vi "Multi_moments_LDA+_An.vi"(3 "Timescales":dbl[](array[numeric]), 4 "Measurement top level?":bool, 6 "Vari Spaced":dbl[][](array[numeric]) format="%.2f") -> (0 "Max Measurement time up":bool, 1 "File info":string[](array[string]), 2 "Vel stat display":string[][](table))   [LabVIEW 2010]
uses:
  Controls/Post_Process.ctl
  Controls/User_Specific_mode.ctl
  Globals/Meas_global.vi
  Globals/Trav_pos_global.vi
  Globals/Dynamic_call_global.ph.vi
  Globals/LDA_meas_global_1.vi
  Acquisition/PWA/PWAtasksGLOBAL.vi
panel:
  out "Sd Error Theshold value":dbl
  out "Instrument Code Name":string
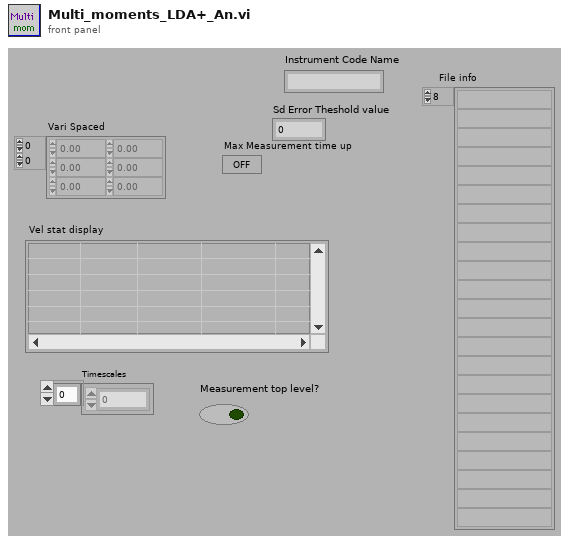
[diagram p1: front panel]
types:
  T1 = typedef "Analysis_info_cluster.ctl" = cluster{"Colour":u32, "Inst type":T2, "Inst name":string, "Symbol":string, "Code name":string, "Extra Info":string, "Inst Array":T3, "Index":i32, "Voltage Index":i32, "Extra Titles":string[], "Extra Values":string[]}
  T2 = typedef "Inst_type.ctl" = enum16{"Propeller anemometer", "Raw voltage", "Pressure Transducer", "Pitot-static tube", "Preston tube", "Hot wire", "Cross wire 1", "Cross wire 2", "Generic Linear", "Generic Polynomial", "Generic BackPoly", "Fast FID", "Thermocouple", "Cold wire", "Pulsed Wire", "LDA Vel", "LDA Tran time", "LDA Arr time"}
  T3 = typedef "Instrument_Array.ctl" = enum16{"PWA", "LDA", "Analogue"}
  T4 = typedef "Post_Process.ctl" = enum16{"Take New Data", "Post Process Raw Data File"}
  T5 = typedef "PWA_Data.ctl" = enum16{"No PWA Data", "One Ch PWA"}
  T6 = typedef "User_Specific_mode.ctl" = enum16{"Check VI only", "Run VI"}
  T7 = cluster{"Name":string, "X":dbl, "Y":dbl, "Z":dbl}[]
  T8 = typedef "Traverse_cluster.ctl" = cluster{"Start X":dbl, "Start Y":dbl, "Start Z":dbl, "End X":dbl, "End Y":dbl, "End Z":dbl, "No. of pts.":i32, "Spacing":T9, "Filename":path, "Tunnel Speed":dbl, "Averaging time (min)":dbl, "Extra Commands":string, "Specific Arguments":string, "Emission Rate (l/min)":dbl, "Trace Gas Concentration (%)":dbl, "Density Ratio":string, "Comments":string, "Row No":i32, "Row Type Selector":T10, "Completion time":string, "Row Duration (mins)":dbl, "No. of Valid pts.":i32, "Meas Setup File":string}
  T9 = typedef "Spacing.ctl" = enum16{"Linear", "Log", "Gauss", "Specified", "N/A"}
  T10 = typedef "Multi_run_mode.ctl" = enum16{"Move Traverse Only", "Set Tunnel Speed Only", "Set Source Only", "Set Measurement Conditions", "Single Measurement", "Vertical Profile", "Lateral Profile", "Longitudinal Profile", "Explore Volume", "Multi-Axis Profile", "Auto Calibrate", "Meas Fast FID Bkgnd", "Check Beam Power", "Scanning Valve Measurement", "Run VI Named:", "Set ADAM Ch", "Wait (minutes)", "Send Message", "Synchronize With:", "Fall Back to this Row", "Turn Off Row Repeating", "Blank Row"}
  T11 = typedef "Velocity_cluster.ctl" = cluster{"Name":string, "U":dbl, "u^2":dbl, "u^3/(u^2)^(1.5)":dbl, "u^4/(u^2)^2 -3":dbl, "% u'/U":dbl, "Mean % Err":dbl, "u^4":dbl}
  T12 = typedef "Correlation_cluster.ctl" = cluster{"U inst":string, "W inst":string, "uw":dbl, "uw/u'w'":dbl, "u^2w":dbl, "uw^2":dbl, "uw^3":dbl, "u^3w":dbl, "u^2w^2":dbl}
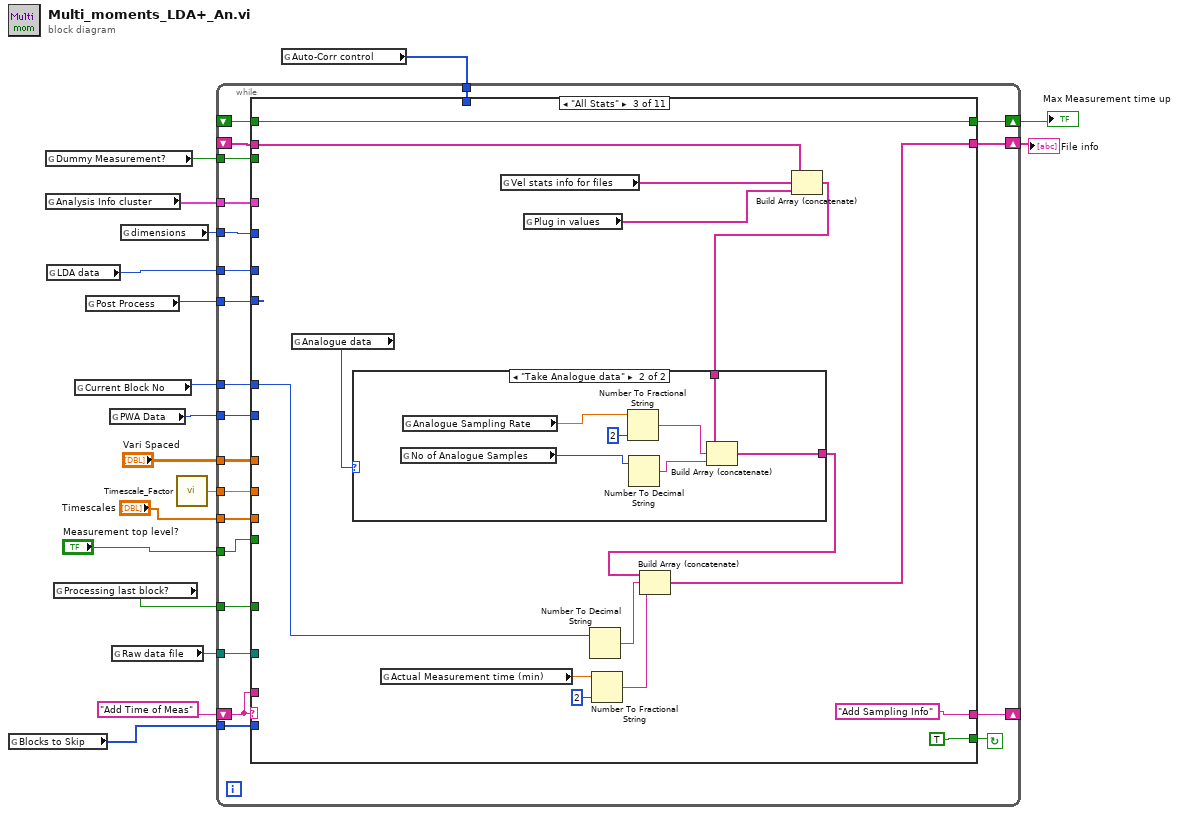
[diagram p0: block diagram]
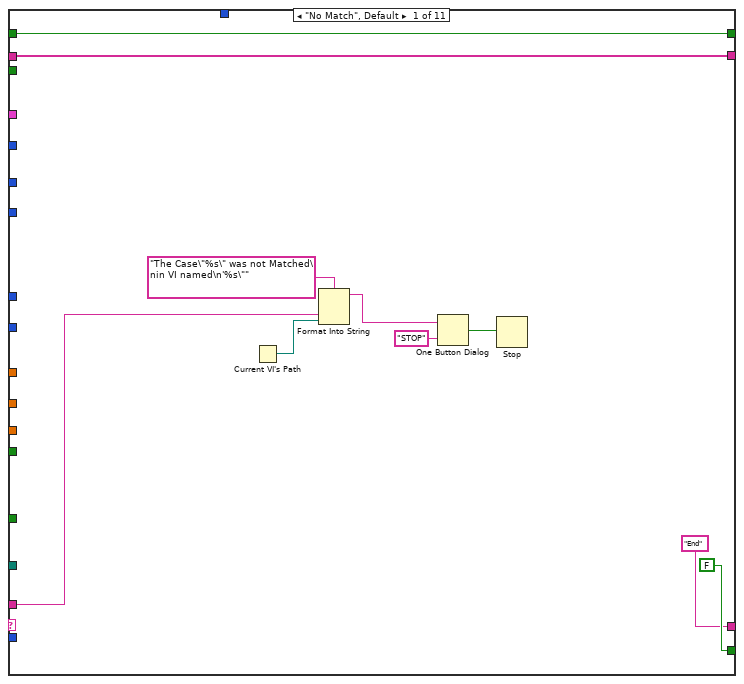
[diagram p2: hidden frame]
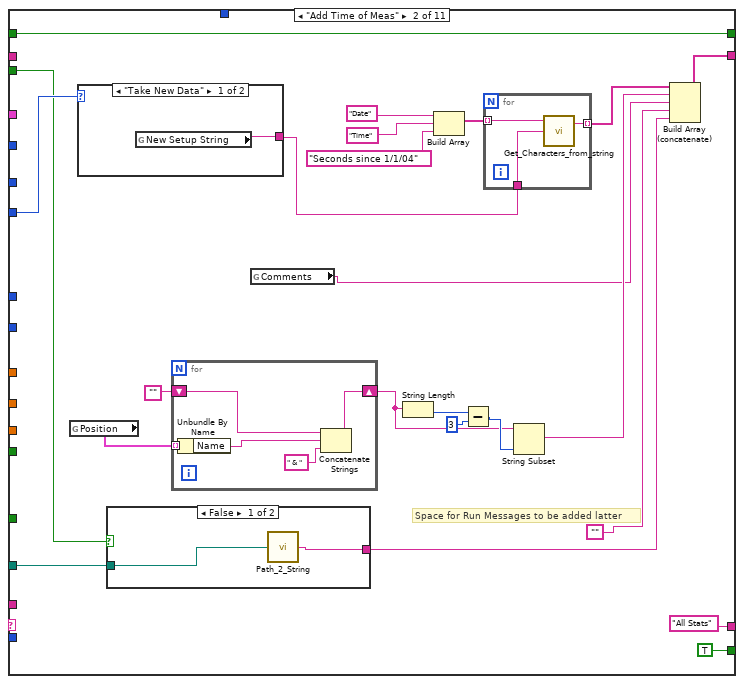
[diagram p3: hidden frame]
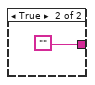
[diagram p4: hidden frame]
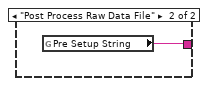
[diagram p5: hidden frame]
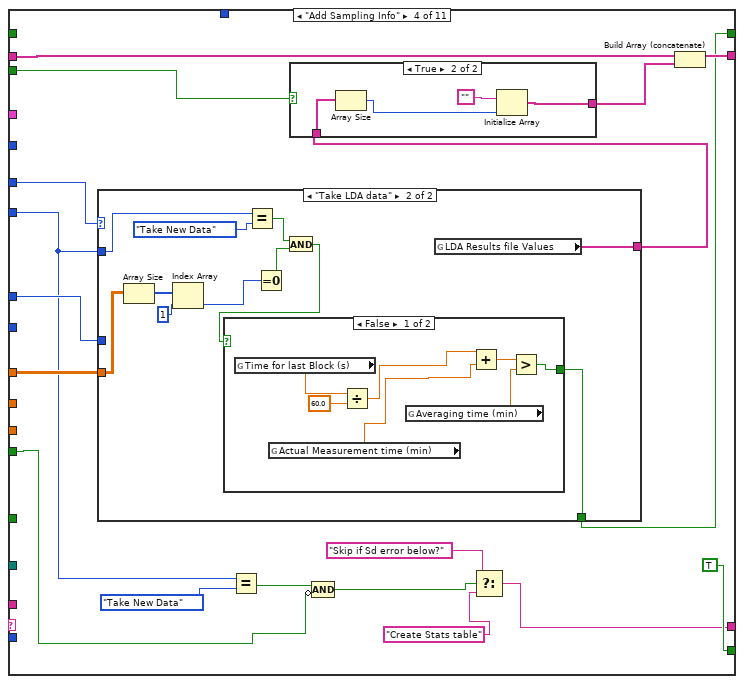
[diagram p7: hidden frame]
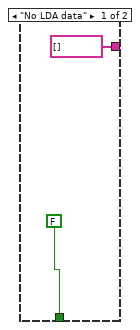
[diagram p9: hidden frame]
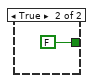
[diagram p10: hidden frame]
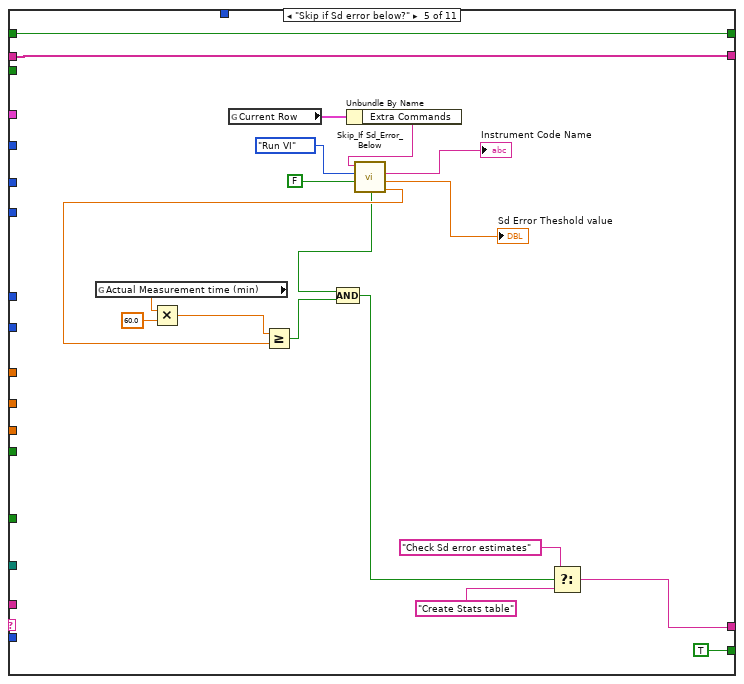
[diagram p11: hidden frame]
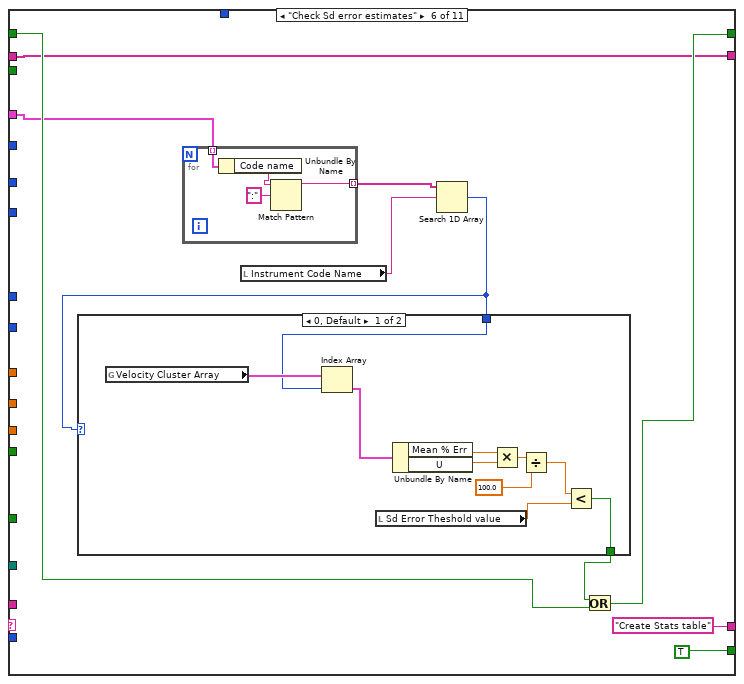
[diagram p12: hidden frame]
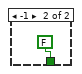
[diagram p13: hidden frame]
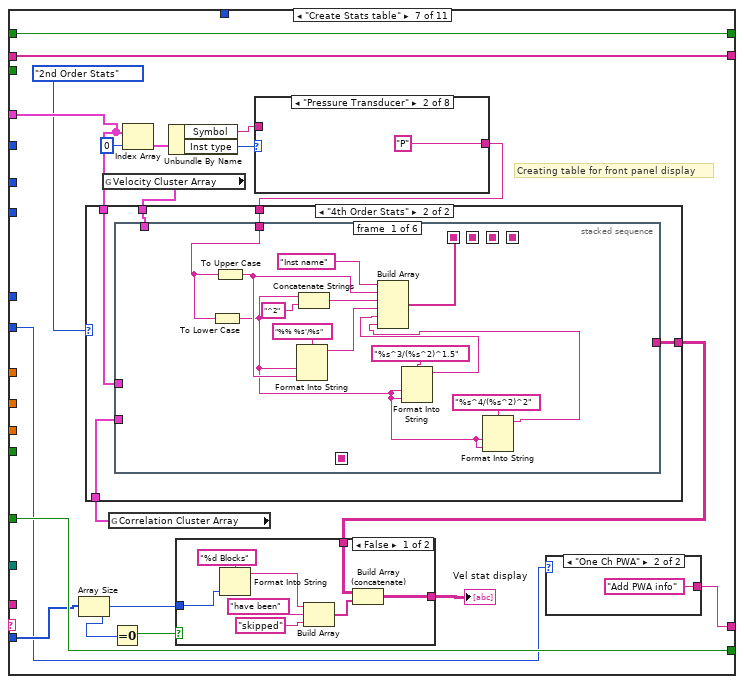
[diagram p14: hidden frame]
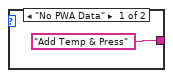
[diagram p15: hidden frame]
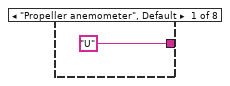
[diagram p17: hidden frame]
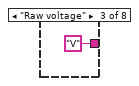
[diagram p18: hidden frame]
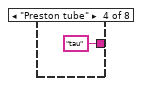
[diagram p19: hidden frame]
diagram:
  n1 = global read "Meas_global.vi" "Blocks to Skip"() -> (w3:i32[])
  n2 = global read "Trav_pos_global.vi" "Dummy Measurement?"() -> (w10:bool)
  n3 = global read "Meas_global.vi" "Analysis Info cluster"() -> (w16:T1[])
  n4 = global read "Meas_global.vi" "LDA data"() -> (w18:enum16{"No LDA data", "Take LDA data"})
  n5 = global read "Meas_global.vi" "Processing last block?"() -> (w12:bool)
  n6 = global read "Meas_global.vi" "Current Block No"() -> (w17:i32)
  n7 = global read "Meas_global.vi" "Post Process"() -> (w15:T4)
  n8 = global read "Meas_global.vi" "PWA Data"() -> (w2:T5)
  n9 = global read "Meas_global.vi" "Raw data file"() -> (w1:path)
  n10 = global read "Meas_global.vi" "dimensions"() -> (w13:enum16{"1D", "2D"})
  n11 = call "Timescale_Factor.vi"() -> ("Factor to scale timescale by"=w4:dbl)
  n12 = global read "Meas_global.vi" "Auto-Corr control"() -> (w7:i32[])
  n13 = while {
    tunnel: "Vari Spaced" -> [w30]
    tunnel: w12 -> [w31]
    tunnel: w13 -> [w32]
    shift-left: _ -> [w33]
    shift-right: [w34] -> w14
    shift-left: "Add Time of Meas" -> [w22]
    shift-right: [w35] -> _
    tunnel: w15 -> [w37]
    tunnel: w16 -> [w38]
    tunnel: w17 -> [w39]
    tunnel: w18 -> [w40]
    tunnel: w10 -> [w29]
    tunnel: "Timescales" -> [w28]
    tunnel: w7 -> [w27]
    shift-right: [w26] -> w6
    shift-left: _ -> [w25]
    tunnel: "Measurement top level?" -> [w24]
    tunnel: w4 -> [w23]
    tunnel: w3 -> [w21]
    tunnel: w2 -> [w20]
    tunnel: w1 -> [w19]
    stop <- w36 continue-if-true
    n14 = case shown="\"All Stats\"" w22 {
      tunnel: w38 -> [_ _ _ _ _ w180 w212 _ _ _ _]
      tunnel: w40 -> [_ _ _ w125 _ _ _ _ _ _ _]
      tunnel: w39 -> [_ _ w89 w124 _ _ _ w393 _ _ _]
      tunnel: w37 -> [_ w55 _ w116 _ _ _ _ w457 w506 w556]
      tunnel: [FALSE ("Processing last block?") TRUE TRUE TRUE ("Processing last block?") TRUE ("Processing last block?") TRUE ("Processing last block?") w208 TRUE ("Processing last block?") TRUE ("Processing last block?") TRUE ("Processing last block?") FALSE] -> w36
      tunnel: ["End" "All Stats" "Add Sampling Info" w114 w157 "Create Stats table" w199 "Add Temp & Press" "Replace Run Messages" "Add Original Results filename" "End"] -> w35
      tunnel: [w42 w72 w87 w126 w162 w176 w215 w396 w466 w509 w553] -> w34
      tunnel: w33 -> [w42 _ w100 w127 w162 w176 w215 w397 w467 w507 w551]
      tunnel: w32 -> [_ _ _ _ _ _ _ _ _ _ _]
      tunnel: w31 -> [_ _ _ _ _ _ w208 _ _ _ _]
      tunnel: w30 -> [_ _ _ w123 _ _ _ _ _ _ _]
      tunnel: w22 -> [w45 _ _ _ _ _ _ _ _ _ _]
      tunnel: w29 -> [_ w54 _ w122 _ _ _ _ _ w497 _]
      tunnel: w28 -> [_ _ _ _ _ _ _ _ _ _ _]
      tunnel: w27 -> [_ _ _ _ _ _ _ _ _ _ _]
      tunnel: [w41 w53 w96 w119 w163 w182 w206 w399 w459 w495 w548] -> w26
      tunnel: w25 -> [w41 w53 w96 _ w163 w181 w206 w399 w459 w495 w548]
      tunnel: w24 -> [_ _ _ w111 _ _ _ _ _ _ _]
      tunnel: w23 -> [_ _ _ _ _ _ _ _ _ _ _]
      tunnel: w21 -> [_ _ _ _ _ _ w204 _ _ w491 _]
      tunnel: w20 -> [_ _ _ _ _ _ w200 _ _ _ _]
      tunnel: w19 -> [_ w51 _ _ _ _ _ _ w456 _ _]
      frame "No Match", Default {
        n15 = Current VI's Path() -> (path=w46:path)
        n16 = Format Into String(format string="The Case\"%s\" was not Matched\nin VI named\n'%s\"" ("Format String"), w45, w46) -> (resulting string=w49:string)  [unwired: 2 in, 1 out]
        n17 = One Button Dialog(message=w49, button name ("OK")="STOP") -> (true=w47:bool)
        n18 = Stop(stop? (T)=w47) -> ()
      }
      frame "Add Time of Meas" {
        # "Space for Run Messages to be added latter"
        n19 = global read "Meas_global.vi" "Position"() -> (w62:T7)
        n20 = case shown="\"Take New Data\"" w55 {
          tunnel: [w85 w86] -> w66
          frame "Take New Data" {
            n21 = global read "Meas_global.vi" "New Setup String"() -> (w85:string)
          }
          frame "Post Process Raw Data File" {
            n22 = global read "Meas_global.vi" "Pre Setup String"() -> (w86:string)
          }
        }
        n23 = case shown="False" w54 {
          tunnel: [w75 ""] -> w64
          tunnel: w51 -> [w74 _]
          frame False {
            n24 = call "Path_2_String.vi"("Real Path"=w74) -> ("Path String"=w75:string)
          }
          frame True {
          }
        }
        n25 = for {
          shift-right: [w80] -> w58
          shift-left: "" -> [w81]
          tunnel: w62 -> [w78] mode=indexing
          n26 = Unbundle By Name(w78) -> ("Name"=w77:string)
          n27 = Concatenate Strings(w81, w77, " & ") -> (w80:string)
        }
        n28 = global read "Meas_global.vi" "Comments"() -> (w52:string)
        n29 = String Length(string=w58) -> (length=w61:i32)
        n30 = Build Array("Date", "Time", "Seconds since 1/1/04") -> (w68:string[])
        n31 = Subtract(x=w61, y=3) -> (x-y=w59:i32)
        n32 = for {
          tunnel: w68 -> [w84] mode=indexing
          tunnel: w66 -> [w83]
          tunnel: [w82] -> w67 mode=indexing
          n33 = call "Get_Characters_from_string.vi"("Input string"=w83, "Variable name"=w84) -> ("Value"=w82:string)  [unwired: 1 in, 1 out]
        }
        n34 = String Subset(string=w58, length (rest)=w59) -> (substring=w56:string)  [unwired: 1 out]
        n35 = Build Array (concatenate)(w67, w56, w52, "", w64) -> (w72:string[])
      }
      frame "All Stats" {
        n36 = global read "Meas_global.vi" "Analogue data"() -> (w95:enum16{"No Analogue data", "Take Analogue data"})
        n37 = global read "Meas_global.vi" "Actual Measurement time (min)"() -> (w90:dbl)
        n38 = global read "Meas_global.vi" "Vel stats info for files"() -> (w97:string[])
        n39 = global read "Dynamic_call_global.ph.vi" "Plug in values"() -> (w99:string[])
        n40 = Number To Decimal String(number=w89) -> (decimal integer string=w93:string)  [unwired: 1 out]
        n41 = Number To Fractional String(number=w90, precision (6)=i16 2) -> (F-format string=w92:string)  [unwired: 2 out]
        n42 = Build Array (concatenate)(w100, w97, w99) -> (w94:string[])
        n43 = case shown="\"Take Analogue data\"" w95 {
          tunnel: w94 -> [w102 w104]
          tunnel: [w102 w103] -> w88
          frame "No Analogue data" {
          }
          frame "Take Analogue data" {
            n44 = global read "Meas_global.vi" "No of Analogue Samples"() -> (w107:i32)
            n45 = global read "Meas_global.vi" "Analogue Sampling Rate"() -> (w108:dbl)
            n46 = Number To Fractional String(number=w108, precision (6)=i16 2) -> (F-format string=w106:string)  [unwired: 2 out]
            n47 = Number To Decimal String(number=w107) -> (decimal integer string=w105:string)  [unwired: 1 out]
            n48 = Build Array (concatenate)(w104, w106, w105) -> (w103:string[])
          }
        }
        n49 = Build Array (concatenate)(w88, w93, w92) -> (w87:string[])
      }
      frame "Add Sampling Info" {
        n50 = case shown="\"Take LDA data\"" w125 {
          tunnel: w124 -> [_ _]
          tunnel: [FALSE w145] -> w119
          tunnel: w116 -> [_ w137]
          tunnel: [string[] [] w135] -> w118
          tunnel: w123 -> [_ w138]
          frame "No LDA data" {
          }
          frame "Take LDA data" {
            n51 = Array Size(array=w138) -> (size(s)=w144:i32[])
            n52 = Index Array(array=w144, index=1 ("Index")) -> (element=w142:i32)
            n53 = Equal?(x=w137, y=Post_Process."Take New Data" ("Post Process")) -> (x = y?=w139:bool)
            n54 = Equal To 0?(x=w142) -> (x = 0?=w140:bool)
            n55 = And(x=w139, y=w140) -> (x .and. y?=w136:bool)
            n56 = case shown="False" w136 {
              tunnel: [w151 FALSE] -> w145
              frame False {
                n57 = global read "LDA_meas_global_1.vi" "Time for last Block (s)"() -> (w149:dbl)
                n58 = global read "Meas_global.vi" "Actual Measurement time (min)"() -> (w146:dbl)
                n59 = Divide(x=w149, y=60.0) -> (x/y=w147:dbl)
                n60 = global read "Meas_global.vi" "Averaging time (min)"() -> (w152:dbl)
                n61 = Add(x=w147, y=w146) -> (x+y=w150:dbl)
                n62 = Greater?(x=w150, y=w152) -> (0:w151:bool)
              }
              frame True {
              }
            }
            n63 = global read "LDA_meas_global_1.vi" "LDA Results file Values"() -> (w135:string[])
          }
        }
        n64 = Equal?(x=w116, y=Post_Process."Take New Data" ("Post Process")) -> (x = y?=w112:bool)
        n65 = case shown="True" w122 {
          tunnel: [w128 w129] -> w121
          tunnel: w118 -> [w128 w132]
          frame False {
          }
          frame True {
            n66 = Array Size(array=w132) -> (size(s)=w131:i32)
            n67 = Initialize Array("", w131) -> (w129:string[])
          }
        }
        n68 = Compound Arithmetic op=AND(w112, invert w111) -> (w110:bool)
        n69 = Select(t="Skip if Sd error below?", s=w110, f="Create Stats table") -> (s? t:f=w114:string)
        n70 = Build Array (concatenate)(w127, w121) -> (w126:string[])
      }
      frame "Skip if Sd error below?" {
        n71 = global read "Meas_global.vi" "Actual Measurement time (min)"() -> (w161:dbl)
        n72 = Multiply(x=w161, y=60.0) -> (x*y=w159:dbl)
        n73 = global read "Trav_pos_global.vi" "Current Row"() -> (w172:T8)
        n74 = Unbundle By Name(w172) -> ("Extra Commands"=w171:string)
        n75 = call "Skip_If Sd_Error_Below.vi"("String to Search"=w171, "Simulate/Run"=User_Specific_mode."Run VI", "Measurement setup Applied?"=FALSE) -> ("Check for Skip?"=w166:bool, "Instrument Code Name"=→"Instrument Code Name":string, "Sd Error Theshold value"=→"Sd Error Theshold value":dbl, "Minimum Measurement time (Sec)"=w168:dbl)  [unwired: 2 in, 1 out]
        n76 = Greater Or Equal?(x=w159, y=w168) -> (x >= y?=w165:bool)
        n77 = Compound Arithmetic op=AND(w166, w165) -> (w154:bool)
        n78 = Select(t="Check Sd error estimates", s=w154, f="Create Stats table") -> (s? t:f=w157:string)
      }
      frame "Check Sd error estimates" {
        n79 = for {
          tunnel: w180 -> [w195] mode=indexing
          tunnel: [w194] -> w179 mode=indexing
          n80 = Unbundle By Name(w195) -> ("Code name"=w197:string)
          n81 = Match Pattern(string=w197, regular expression=":") -> (before substring=w194:string)  [unwired: 4 out]
        }
        n82 = local read "Instrument Code Name"() -> (w178:string)
        n83 = Search 1D Array(1D array=w179, element=w178) -> (index of element=w173:i32)  [unwired: 1 out]
        n84 = case shown="0, Default" w173 {
          tunnel: w173 -> [w191 _]
          tunnel: [w183 FALSE] -> w177
          frame 0, Default {
            n85 = global read "Meas_global.vi" "Velocity Cluster Array"() -> (w192:T11[])
            n86 = Index Array(array=w192, index=w191) -> (element=w190:T11)
            n87 = local read "Sd Error Theshold value"() -> (w184:dbl)
            n88 = Unbundle By Name(w190) -> ("Mean % Err"=w189:dbl, "U"=w188:dbl)
            n89 = Multiply(x=w189, y=w188) -> (x*y=w187:dbl)
            n90 = Divide(x=w187, y=100.0) -> (x/y=w185:dbl)
            n91 = Less?(x=w185, y=w184) -> (x < y?=w183:bool)
          }
          frame -1 {
          }
        }
        n92 = Or(x=w177, y=w181) -> (x .or. y?=w182:bool)
      }
      frame "Create Stats table" {
        # "Creating table for front panel display"
        n93 = Array Size(array=w204) -> (size(s)=w202:i32)
        n94 = global read "Meas_global.vi" "Velocity Cluster Array"() -> (w207:T11[])
        n95 = global read "Meas_global.vi" "Correlation Cluster Array"() -> (w216:T12[])
        n96 = Equal To 0?(x=w202) -> (x = 0?=w201:bool)
        n97 = Index Array(array=w212, index=0) -> (element=w214:T1)
        n98 = Unbundle By Name(w214) -> ("Symbol"=w210:string, "Inst type"=w211:T2)
        n99 = case shown="\"Pressure Transducer\"" w211 {
          tunnel: ["U" "P" "V" "tau" w232 "C" ("Symbol") "T" ("Symbol") "T" ("Symbol")] -> w209
          tunnel: w210 -> [_ _ _ _ w232 _ _ _]
          frame "Propeller anemometer", Default {
          }
          frame "Pressure Transducer" {
          }
          frame "Raw voltage" {
          }
          frame "Preston tube" {
          }
          frame "Generic Linear" {
          }
          frame "Fast FID" {
          }
          frame "Thermocouple" {
          }
          frame "Cold wire" {
          }
        }
        n100 = case shown="\"4th Order Stats\"" enum16{"2nd Order Stats", "4th Order Stats"}."2nd Order Stats" ("Mode selector") {
          tunnel: w212 -> [w240 w311]
          tunnel: [w239 w310] -> w205
          tunnel: w207 -> [w238 w309]
          tunnel: w216 -> [w237 w308]
          tunnel: w209 -> [w236 w307]
          frame "2nd Order Stats" {
            n101 = stacked-sequence {
              seq-local: [w244 _ _ _ _ _] -> [_ _ _ _ _ w305]
              seq-local: [_ _ w275 _ _ _] -> [_ _ _ _ _ w304]
              seq-local: [_ _ _ w284 _ _] -> [_ _ _ _ _ w303]
              seq-local: [_ _ _ _ w292 _] -> [_ _ _ _ _ w302]
              seq-local: [_ w253 _ _ _ _] -> [_ _ w276 _ _ _]
              tunnel: w240 -> [_ _ w277 _ _ _]
              tunnel: [_ _ _ _ _ w306] -> w239
              tunnel: w238 -> [_ w252 _ _ _ _]
              tunnel: w237 -> [_ _ _ w282 w291 _]
              tunnel: w236 -> [w243 _ _ _ _ _]
              frame #0 {
                n102 = To Lower Case(string=w243) -> (all lower case string=w248:string)
                n103 = To Upper Case(1:w243) -> (0:w246:string)
                n104 = Format Into String(format string="%% %s'/%s", w248, w246) -> (resulting string=w247:string)  [unwired: 2 in, 1 out]
                n105 = Concatenate Strings(w248, "^2") -> (w250:string)
                n106 = Build Array("Inst name", w246, w250, w247, "Sd Err in Mean", "% Sd Err") -> (w244:string[])
              }
              frame #1 {
                n107 = for {
                  tunnel: [w269] -> _ mode=indexing
                  tunnel: [w268] -> w253 mode=indexing
                  tunnel: w252 -> [w269] mode=indexing
                  n108 = Unbundle By Name(w269) -> ("U"=w256:dbl, "u^2"=w263:dbl, "% u'/U"=w266:dbl, "Mean % Err"=w258:dbl)
                  n109 = Compound Arithmetic op=MULTIPLY(w256, 0.01 ("value"), w258) -> (w255:dbl)
                  n110 = call "Number_2_string.vi"("number"=w255) -> ("String"=w254:string)  [unwired: 1 in]
                  n111 = call "Number_2_string.vi"("number"=w263) -> ("String"=w262:string)  [unwired: 1 in]
                  n112 = call "Number_2_string.vi"("number"=w256) -> ("String"=w261:string)  [unwired: 1 in]
                  n113 = Number To Fractional String(number=w266, precision (6)=i16 2) -> (F-format string=w265:string)  [unwired: 2 out]
                  n114 = Number To Fractional String(number=w258, precision (6)=i16 2) -> (F-format string=w259:string)  [unwired: 2 out]
                  n115 = Build Array(w261, w262, w265, w254, w259) -> (w264:string[])
                  n116 = for {
                    tunnel: [w273] -> w268 mode=indexing
                    tunnel: w264 -> [w270] mode=indexing
                    n117 = Equal?(x="NaN", y=w270) -> (x = y?=w274:bool)
                    n118 = Select(t="", s=w274, f=w270) -> (s? t:f=w273:string)
                  }
                }
              }
              frame #2 {
                n119 = for {
                  tunnel: w277 -> [w281] mode=indexing
                  tunnel: w276 -> [w279] mode=indexing
                  tunnel: [w278] -> w275 mode=indexing
                  n120 = Unbundle By Name(w281) -> ("Inst name"=w280:string)
                  n121 = Build Array (concatenate)(w280, w279) -> (w278:string[])
                }
              }
              frame #3 {
                n122 = Array Size(array=w282) -> (size(s)=w283:i32)
                n123 = case shown="0" w283 {
                  tunnel: [string[] [] w286] -> w284
                  frame 0 {
                  }
                  frame 1, Default {
                    n124 = Build Array("u inst", "w inst", "uw", "uw/u'w'") -> (w286:string[])
                  }
                }
              }
              frame #4 {
                n125 = for {
                  tunnel: [w299] -> w292 mode=indexing
                  tunnel: w291 -> [w298] mode=indexing
                  n126 = Unbundle By Name(w298) -> ("U inst"=w301:string, "W inst"=w300:string, "uw"=w294:dbl, "uw/u'w'"=w296:dbl)
                  n127 = call "Number_2_string.vi"("number"=w294) -> ("String"=w293:string)  [unwired: 1 in]
                  n128 = Number To Fractional String(number=w296, precision (6)=i16 3) -> (F-format string=w295:string)  [unwired: 2 out]
                  n129 = Build Array(w301, w300, w293, w295) -> (w299:string[])
                }
              }
              frame #5 {
                n130 = Build Array (concatenate)(w305, w304, w303, w302) -> (w306:string[][])
              }
            }
          }
          frame "4th Order Stats" {
            n131 = stacked-sequence {
              seq-local: [w312 _ _ _ _ _] -> [_ _ _ _ _ w384]
              seq-local: [_ _ w348 _ _ _] -> [_ _ _ _ _ w383]
              seq-local: [_ _ _ w357 _ _] -> [_ _ _ _ _ w382]
              seq-local: [_ _ _ _ w367 _] -> [_ _ _ _ _ w381]
              seq-local: [_ w326 _ _ _ _] -> [_ _ w349 _ _ _]
              tunnel: w311 -> [_ _ w350 _ _ _]
              tunnel: [_ _ _ _ _ w385] -> w310
              tunnel: w309 -> [_ w325 _ _ _ _]
              tunnel: w308 -> [_ _ _ w355 w366 _]
              tunnel: w307 -> [w317 _ _ _ _ _]
              frame #0 {
                n132 = To Lower Case(string=w317) -> (all lower case string=w316:string)
                n133 = To Upper Case(1:w317) -> (0:w320:string)
                n134 = Format Into String(format string="%% %s'/%s", w316, w320) -> (resulting string=w321:string)  [unwired: 2 in, 1 out]
                n135 = Concatenate Strings(w316, "^2") -> (w323:string)
                n136 = Format Into String(format string="%s^3/(%s^2)^1.5", w316, w316) -> (resulting string=w315:string)  [unwired: 2 in, 1 out]
                n137 = Format Into String(format string="%s^4/(%s^2)^2", w316, w316) -> (resulting string=w314:string)  [unwired: 2 in, 1 out]
                n138 = Build Array("Inst name", w320, w323, w321, w315, w314) -> (w312:string[])
              }
              frame #1 {
                n139 = for {
                  tunnel: [w342] -> _ mode=indexing
                  tunnel: [w340] -> w326 mode=indexing
                  tunnel: w325 -> [w342] mode=indexing
                  n140 = Unbundle By Name(w342) -> ("U"=w329:dbl, "u^2"=w341:dbl, "% u'/U"=w335:dbl, "u^3/(u^2)^(1.5)"=w337:dbl, "u^4/(u^2)^2 -3"=w334:dbl)
                  n141 = Number To Fractional String(number=w335, precision (6)=i16 2) -> (F-format string=w333:string)  [unwired: 2 out]
                  n142 = call "Number_2_string.vi"("number"=w341) -> ("String"=w328:string)  [unwired: 1 in]
                  n143 = Number To Fractional String(number=w337, precision (6)=i16 3) -> (F-format string=w332:string)  [unwired: 2 out]
                  n144 = Number To Fractional String(number=w334, precision (6)=i16 3) -> (F-format string=w331:string)  [unwired: 2 out]
                  n145 = call "Number_2_string.vi"("number"=w329) -> ("String"=w327:string)  [unwired: 1 in]
                  n146 = Build Array(w327, w328, w333, w332, w331) -> (w330:string[])
                  n147 = for {
                    tunnel: [w346] -> w340 mode=indexing
                    tunnel: w330 -> [w343] mode=indexing
                    n148 = Equal?(x="NaN", y=w343) -> (x = y?=w347:bool)
                    n149 = Select(t="", s=w347, f=w343) -> (s? t:f=w346:string)
                  }
                }
              }
              frame #2 {
                n150 = for {
                  tunnel: w350 -> [w354] mode=indexing
                  tunnel: w349 -> [w352] mode=indexing
                  tunnel: [w351] -> w348 mode=indexing
                  n151 = Unbundle By Name(w354) -> ("Inst name"=w353:string)
                  n152 = Build Array (concatenate)(w353, w352) -> (w351:string[])
                }
              }
              frame #3 {
                n153 = Array Size(array=w355) -> (size(s)=w356:i32)
                n154 = case shown="..0" w356 {
                  tunnel: [string[] [] w364] -> w357
                  frame ..0 {
                  }
                  frame 1.. {
                    n155 = Build Array("u inst", "w inst", "uw", "uw/u'w'", "u^2w", "uw^2") -> (w364:string[])
                  }
                }
              }
              frame #4 {
                n156 = for {
                  tunnel: [w380] -> w367 mode=indexing
                  tunnel: w366 -> [w379] mode=indexing
                  (unwired) i16 3 ("precision (6)")
                  n157 = Unbundle By Name(w379) -> ("U inst"=w378:string, "W inst"=w377:string, "uw"=w369:dbl, "uw/u'w'"=w374:dbl, "u^2w"=w372:dbl, "uw^2"=w373:dbl)
                  n158 = Number To Fractional String(number=w374, precision (6)=i16 3) -> (F-format string=w375:string)  [unwired: 2 out]
                  n159 = call "Number_2_string.vi"("number"=w369) -> ("String"=w368:string)  [unwired: 1 in]
                  n160 = call "Number_2_string.vi"("number"=w373) -> ("String"=w370:string)  [unwired: 1 in]
                  n161 = call "Number_2_string.vi"("number"=w372) -> ("String"=w371:string)  [unwired: 1 in]
                  n162 = Build Array(w378, w377, w368, w375, w371, w370) -> (w380:string[])
                }
              }
              frame #5 {
                n163 = Build Array (concatenate)(w384, w383, w382, w381) -> (w385:string[][])
              }
            }
          }
        }
        n164 = case shown="False" w201 {
          tunnel: w205 -> [w226 w227]
          tunnel: [w222 w227] -> w203
          tunnel: w202 -> [w221 _]
          frame False {
            n165 = Format Into String(format string="%d Blocks", w221) -> (resulting string=w219:string)  [unwired: 2 in, 1 out]
            n166 = Build Array(w219, "have been" ("element"), "skipped" ("element")) -> (w223:string[])
            n167 = Build Array (concatenate)(w226, w223) -> (w222:string[][])
          }
          frame True {
          }
        }
        "Vel stat display" <- w203
        n168 = case shown="\"One Ch PWA\"" w200 {
          tunnel: ["Add Temp & Press" "Add PWA info"] -> w199
          frame "No PWA Data" {
          }
          frame "One Ch PWA" {
          }
        }
      }
      frame "Add PWA info" {
        n169 = stacked-sequence {
          tunnel: [w430 _] -> w395
          tunnel: [w428 _] -> w394
          tunnel: w393 -> [w426 _]
          tunnel: [w421 _] -> w392
          tunnel: [w416 _] -> w391
          tunnel: [w415 _] -> w390
          tunnel: [_ w433] -> w389
          tunnel: [_ w432] -> w388
          tunnel: [w409 _] -> w387
          tunnel: [w401 _] -> w386
          frame #0 {
            n170 = global read "PWAtasksGLOBAL.vi" "PWA No. of Samples"() -> (w427:i32)
            n171 = global read "PWAtasksGLOBAL.vi" "PWA Freq. (Hz)"() -> (w431:dbl)
            n172 = global read "PWAtasksGLOBAL.vi" "PWA No of  TOF Timeouts"() -> (w406:i32)
            n173 = global read "PWAtasksGLOBAL.vi" "PWA No of  TOF Below Min"() -> (w407:i32)
            n174 = Multiply(x=w427, y=w426) -> (x*y=w408:i32)
            n175 = global read "PWAtasksGLOBAL.vi" "PWA Seconds per clock pulse"() -> (w413:dbl)
            n176 = global read "PWAtasksGLOBAL.vi" "PWA Setup summary"() -> (w415:string)
            n177 = Compound Arithmetic op=ADD(w408, invert w407, invert w406) -> (w404:i32)
            n178 = global read "PWAtasksGLOBAL.vi" "PWA No of Reverse samples"() -> (w405:i32)
            n179 = Number To Fractional String(number=w431, precision (6)=i16 2) -> (F-format string=w430:string)  [unwired: 2 out]
            n180 = Number To Decimal String(number=w427) -> (decimal integer string=w428:string)  [unwired: 1 out]
            n181 = global read "PWAtasksGLOBAL.vi" "Minimum TOF Index"() -> (w414:i16)
            n182 = Divide(x=w406, y=w408) -> (x/y=w425:dbl)
            n183 = Divide(x=w407, y=w408) -> (x/y=w417:dbl)
            n184 = Multiply(x=w425, y=100.0) -> (x*y=w422:dbl)
            n185 = Multiply(x=w417, y=100.0) -> (x*y=w420:dbl)
            n186 = Number To Fractional String(number=w422, precision (6)=i16 2) -> (F-format string=w421:string)  [unwired: 2 out]
            n187 = Number To Fractional String(number=w420, precision (6)=i16 2) -> (F-format string=w416:string)  [unwired: 2 out]
            n188 = Multiply(x=w413, y=w414) -> (x*y=w412:dbl)
            n189 = Divide(x=w405, y=w404) -> (x/y=w402:dbl)
            n190 = Multiply(x=w412, y=1000000.0) -> (x*y=w410:dbl)
            n191 = Number To Fractional String(number=w402, precision (6)=i16 6) -> (F-format string=w401:string)  [unwired: 2 out]
            n192 = Number To Decimal String(number=w410) -> (decimal integer string=w409:string)  [unwired: 1 out]
          }
          frame #1 {
            w446 = 4095
            w442 = 4095
            n193 = global read "PWAtasksGLOBAL.vi" "Minimum TOF Index"() -> (w441:i16)
            n194 = global read "PWAtasksGLOBAL.vi" "PWA Lookup Table"() -> (w445:dbl[])
            n195 = Negate(x=w442) -> (-x=w444:i32)
            n196 = Negate(x=w441) -> (-x=w443:i16)
            n197 = Add(x=w442, y=w446) -> (x+y=w447:i32)
            n198 = Add(x=w441, y=w446) -> (x+y=w448:i32)
            n199 = Add(x=w443, y=w446) -> (x+y=w450:i32)
            n200 = Add(x=w444, y=w446) -> (x+y=w449:i32)
            n201 = Index Array(array=w445, index=w447) -> (element=w440:dbl)
            n202 = Index Array(array=w445, index=w448) -> (element=w439:dbl)
            n203 = Index Array(array=w445, index=w449) -> (element=w436:dbl)
            n204 = Index Array(array=w445, index=w450) -> (element=w434:dbl)
            n205 = global read "PWAtasksGLOBAL.vi" "PWA Symbol"() -> (w435:string)
            n206 = Format Into String(format string="%.3f<%s<%.2f", w440, w435, w439) -> (resulting string=w433:string)  [unwired: 2 in, 1 out]
            n207 = Format Into String(format string=" %.3f<%s<%.2f", w436, w435, w434) -> (resulting string=w432:string)  [unwired: 2 in, 1 out]
          }
        }
        n208 = Build Array (concatenate)(w397, w395, w394, w387, w392, w391, w390, w386, w389, w388) -> (w396:string[])
      }
      frame "Add Temp & Press" {
        n209 = global read "Meas_global.vi" "Synchronise with LDA"() -> (w454:bool)
        n210 = case shown="\"Post Process Raw Data File\"" w457 {
          tunnel: [w474 w479] -> w458
          tunnel: w456 -> [_ w485]
          frame "Take New Data" {
            n211 = global read "Meas_global.vi" "Start Time of experiment"() -> (w478:dbl)
            n212 = call "Sec_to_date_filename.vi"("seconds"=w478) -> ("Day"=w476:string, "Time"=w477:string)  [unwired: 2 out]
            n213 = Format Into String(format string="%s on %s", w477, w476) -> (resulting string=w474:string)  [unwired: 2 in, 1 out]
          }
          frame "Post Process Raw Data File" {
            n214 = call "Read_RD_Ch_header.vi"("Raw data file"=w485) -> ("Ch Name Out"=w484:string[], "Ch Values"=w480:string[])  [unwired: 2 out]
            n215 = Search 1D Array(1D array=w484, element="Multi Run:Start Time:") -> (index of element=w481:i32)  [unwired: 1 out]
            n216 = Greater Or Equal To 0?(x=w481) -> (x >= 0?=w482:bool)
            n217 = case shown="True" w482 {
              tunnel: w481 -> [_ w489]
              tunnel: w480 -> [_ w488]
              tunnel: ["" w487] -> w479
              frame False {
              }
              frame True {
                n218 = Index Array(array=w488, index=w489) -> (element=w487:string)
              }
            }
          }
        }
        n219 = global read "Meas_global.vi" "Abs Press (mbar)"() -> (w464:dbl)
        n220 = global read "Meas_global.vi" "Temp"() -> (w460:dbl)
        n221 = Number To Fractional String(number=w464, precision (6)=i16 2) -> (F-format string=w465:string)  [unwired: 2 out]
        n222 = Number To Fractional String(number=w460, precision (6)=i16 1) -> (F-format string=w462:string)  [unwired: 2 out]
        n223 = Build Array(w462, w465, w458) -> (w452:string[])
        n224 = case shown="False" w454 {
          tunnel: w452 -> [w468 w471]
          tunnel: [w468 w469] -> w451
          frame False {
          }
          frame True {
            n225 = global read "LDA_meas_global_1.vi" "Sync Delay Time (ms)"() -> (w472:dbl)
            n226 = Number To Fractional String(number=w472, precision (6)=i16 1) -> (F-format string=w470:string)  [unwired: 2 out]
            n227 = Build Array (concatenate)(w471, w470) -> (w469:string[])
          }
        }
        n228 = Build Array (concatenate)(w467, w451) -> (w466:string[])
      }
      frame "Replace Run Messages" {
        n229 = Array Size(array=w491) -> (size(s)=w492:i32)
        n230 = case shown="\"Take New Data\"" w506 {
          tunnel: ["Take New Data" "Post Process"] -> w505
          frame "Take New Data" {
          }
          frame "Post Process Raw Data File" {
          }
        }
        n231 = global read "Meas_global.vi" "BSA data rate string"() -> (w511:string)
        n232 = global read "Meas_global.vi" "Over/Under string"() -> (w513:string)
        n233 = Equal To 0?(x=w492) -> (x = 0?=w490:bool)
        n234 = global read "Meas_global.vi" "Extra Comments"() -> (w512:string)
        n235 = Concatenate Strings(w511, w513, w512) -> (w510:string)
        n236 = call "Remove_unprintable_Char.vi"("Input String"=w510) -> ("Output String"=w494:string)
        n237 = case shown="False" w490 {
          tunnel: w491 -> [w519 _]
          tunnel: w494 -> [w515 w524]
          tunnel: [w514 w524] -> w493
          frame False {
            n238 = for {
              shift-right: [w521] -> w517
              shift-left: "Blocks " -> [w523]
              tunnel: w519 -> [w522] mode=indexing
              n239 = Format Into String(format string="%d; ", initial string=w523, w522) -> (resulting string=w521:string)  [unwired: 1 in, 1 out]
            }
            n240 = Concatenate Strings(w515, w517, "have been skipped. " ("string")) -> (w514:string)
          }
          frame True {
          }
        }
        n241 = case shown="False" w497 {
          tunnel: [w525 "Dummy Measurement"] -> w496
          tunnel: w493 -> [w525 _]
          frame False {
          }
          frame True {
          }
        }
        n242 = Build Array (concatenate)(w507, w505) -> (w502:string[])
        n243 = for {
          N: 3 -> [_]
          shift-right: [w529] -> w501
          shift-left: w502 -> [w530]
          i -> [w533]
          n244 = case shown="2" w533 {
            tunnel: [w539 w540 w541] -> w527
            frame 0, Default {
              n245 = global read "Dynamic_call_global.ph.vi" "Initial Plug Ins"() -> (w539:string[])
            }
            frame 1 {
              n246 = global read "Dynamic_call_global.ph.vi" "Per Block Plug Ins"() -> (w540:string[])
            }
            frame 2 {
              n247 = global read "Dynamic_call_global.ph.vi" "Final Plug Ins"() -> (w541:string[])
            }
          }
          n248 = Array Size(array=w527) -> (size(s)=w532:i32)
          n249 = for {
            tunnel: w527 -> [w542] mode=indexing
            shift-right: [w543] -> w528
            shift-left: "" -> [w545]
            n250 = Concatenate Strings(w545, w542, ";" ("string")) -> (w543:string)
          }
          n251 = Greater Than 0?(x=w532) -> (x > 0?=w531:bool)
          n252 = case shown="True" w531 {
            tunnel: w530 -> [w535 w538]
            tunnel: [w535 w537] -> w529
            tunnel: w528 -> [_ w536]
            frame False {
            }
            frame True {
              n253 = Build Array (concatenate)(w538, w536) -> (w537:string[])
            }
          }
        }
        n254 = call "First_column_names.vi"() -> ("Array"=w500:string[])
        n255 = Search 1D Array(1D array=w500, element="Run:Messages::") -> (index of element=w499:i32)  [unwired: 1 out]
        n256 = Replace Array Subset(array=w501, new element=w496, index=w499) -> (w509:string[])
      }
      frame "Add Original Results filename" {
        n257 = Equal?(x=w556, y=Post_Process."Take New Data" ("Post Process")) -> (x = y?=w555:bool)
        n258 = case shown="False" w555 {
          tunnel: [w558 w562] -> w550
          frame False {
            n259 = global read "Meas_global.vi" "Pre Setup String"() -> (w561:string)
            n260 = call "Get_Characters_from_string.vi"("Input string"=w561, "Variable name"="Results filename") -> ("Value"=w559:string)  [unwired: 1 in, 1 out]
            n261 = call "String_to_Pathname.vi"("Input String"=w559) -> ("path"=w558:path)
          }
          frame True {
            n262 = global read "Meas_global.vi" "Results file"() -> (w562:path)
          }
        }
        n263 = Strip Path(path=w550) -> (name=w549:string)  [unwired: 1 out]
        n264 = Build Array (concatenate)(w551, w549) -> (w553:string[])
      }
    }
  }
  "File info" <- w14
  "Max Measurement time up" <- w6
